vi "direccion.vi"(9 "Array":string[](array[string]), 10 "String":string) -> (0 "DERECHA":bool, 1 "IZQUIERDA":bool, 2 "ABAJO":bool, 3 "ARRIBA":bool)   [LabVIEW 2016]
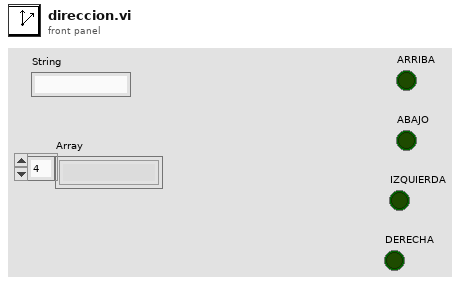
[diagram p1: front panel]
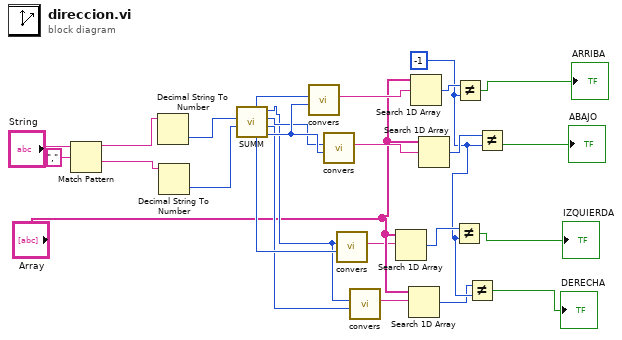
[diagram p0: block diagram]
diagram:
  w4 = -1
  n1 = Match Pattern(string="String", regular expression=",") -> (before substring=w24:string, after substring=w23:string)  [unwired: 1 in, 2 out]
  n2 = Decimal String To Number(string=w24) -> (number=w21:i32)  [unwired: 2 in, 1 out]
  n3 = Decimal String To Number(string=w23) -> (number=w22:i32)  [unwired: 2 in, 1 out]
  n4 = call "SUMM.vi"("Y"=w22, "X"=w21) -> ("Y"=w16:i32, "Y+1"=w8:i32, "X+1"=w15:i32, "X"=w9:i32, "Y-1"=w11:i32, "X-1"=w19:i32)  [unwired: 4 in]
  n5 = call "convers.vi"("Y"=w16, "x"=w19) -> ("salida"=w20:string)  [unwired: 9 in]
  n6 = call "convers.vi"("Y"=w16, "x"=w15) -> ("salida"=w12:string)  [unwired: 9 in]
  n7 = call "convers.vi"("Y"=w11, "x"=w9) -> ("salida"=w5:string)  [unwired: 9 in]
  n8 = call "convers.vi"("Y"=w8, "x"=w9) -> ("salida"=w7:string)  [unwired: 9 in]
  n9 = Search 1D Array(1D array="Array", element=w5) -> (index of element=w10:i32)  [unwired: 1 in]
  n10 = Search 1D Array(1D array="Array", element=w7) -> (index of element=w3:i32)  [unwired: 1 in]
  n11 = Search 1D Array(1D array="Array", element=w20) -> (index of element=w18:i32)  [unwired: 1 in]
  n12 = Search 1D Array(1D array="Array", element=w12) -> (index of element=w13:i32)  [unwired: 1 in]
  n13 = Not Equal?(x=w10, y=w4) -> (x != y?=→"IZQUIERDA":bool)
  n14 = Not Equal?(x=w18, y=w4) -> (x != y?=→"ARRIBA":bool)
  n15 = Not Equal?(x=w3, y=w4) -> (x != y?=→"DERECHA":bool)
  n16 = Not Equal?(x=w13, y=w4) -> (x != y?=→"ABAJO":bool)
